vi "Impedance Excel Export.vi"(0 "template Path":path=path "C:/Users/L025200.LUXSHARE/Desktop/Released VNA Automatic 20150329/Templete/QSFP+_IBM.xls", 1 "Data Basic Path":path=path "S:/PNA_DATA/QSFP+  IBM 3m/Sample_#1_150331", 3 "Sheet Index List":i32[](array[numeric])=[1, 2, 3], 5 "Report  Path":path=path "S:/PNA_DATA/QSFP+  IBM 3m/Sample_#1_150331", 7 "error in (no error)":errorcluster caption="错误输入（无错误）") -> ()   [LabVIEW 2011]
uses:
  <vilib>/Utility/NIReport.llb/NI_report.lvclass
  <vilib>/Utility/file.llb/Read From Spreadsheet File (DBL).vi
  <vilib>/addons/_office/excel.llb/Excel Easy Table (num).vi
  <vilib>/Utility/NIReport.llb/Excel/NI_Excel.lvclass
  <vilib>/addons/_office/NI_ReportGenerationToolkit.lvlib
panel:
  in  "File Name":string=".txt"
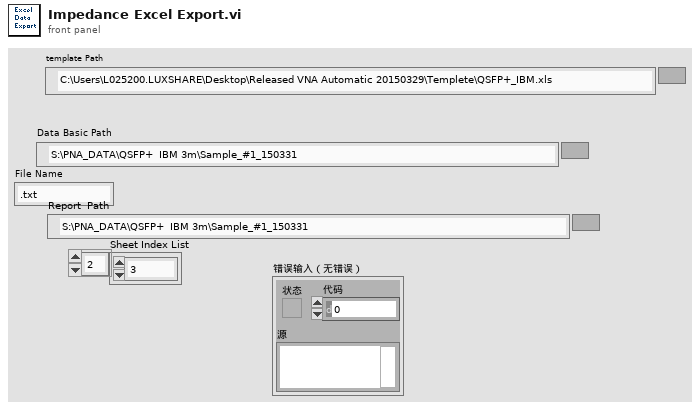
[diagram p1: front panel]
types:
  T1 = enum16{"Standard Report", "HTML", "Word", "Excel"}
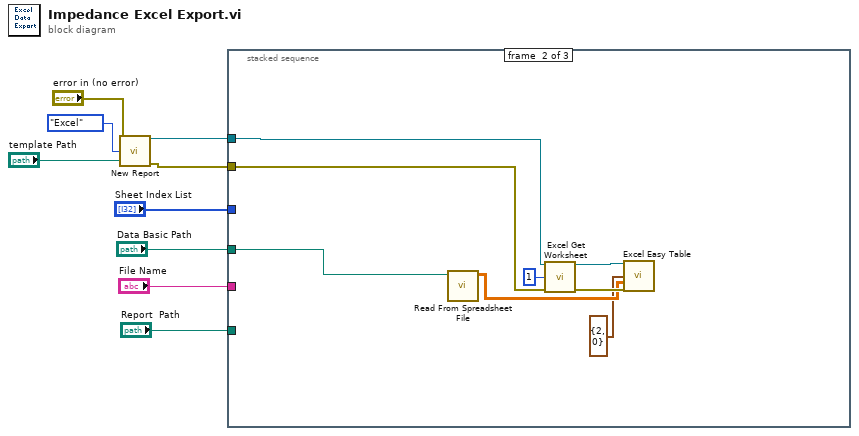
[diagram p0: block diagram]
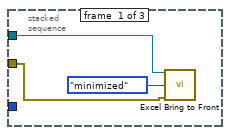
[diagram p2: hidden frame]
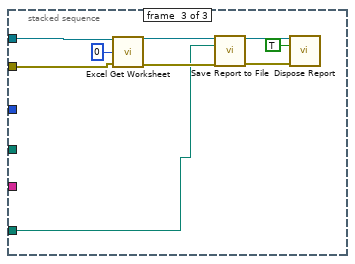
[diagram p3: hidden frame]
diagram:
  n1 = call <vilib>:"New Report.vi"("report type"=T1."Excel", "template (empty)"="template Path", "error in (no error)"="error in (no error)") -> ("report out"=w5:refnum<class "NI_report.lvclass">, "error out"=w3:errorcluster)  [unwired: 11 in]
  n2 = stacked-sequence {
    tunnel: "Data Basic Path" -> [_ w13 _]
    tunnel: "Sheet Index List" -> [_ _ _]
    tunnel: w5 -> [w11 w20 w29]
    tunnel: w3 -> [w10 w19 w22]
    tunnel: "File Name" -> [_ _ _]
    tunnel: "Report  Path" -> [_ _ w21]
    frame #0 {
      n3 = call <vilib>:"Excel Bring to Front.vi"("report in"=w11, "window state (maximized)"=enum16{"maximized", "minimized", "normal"}."minimized", "error in (no error)"=w10) -> ()  [unwired: 11 in, 2 out]
    }
    frame #1 {
      n4 = call-poly <vilib>:"Read From Spreadsheet File.vi"("file path (dialog if empty)"=w13) -> ("all rows"=w15:dbl[][])  [unwired: 6 in, 4 out]
      n5 = call <vilib>:"Excel Get Worksheet.vi"("report in"=w20, "worksheet index (0)"=1, "error in (no error)"=w19) -> ("report out"=w17:refnum<class "NI_report.lvclass">, "error out"=w18:errorcluster)  [unwired: 11 in]
      n6 = call-poly <vilib>:"Excel Easy Table.vi"("report in"=w17, "start (0, 0)"=cluster{"row":i32, "column":i32} {"row"=2, "column"=0}, "text data"=w15, "error in (no error)"=w18) -> ()  [unwired: 7 in, 5 out]
    }
    frame #2 {
      n7 = call <vilib>:"Excel Get Worksheet.vi"("report in"=w29, "worksheet index (0)"=0, "error in (no error)"=w22) -> ("report out"=w23:refnum<class "NI_report.lvclass">, "error out"=w24:errorcluster)  [unwired: 11 in]
      n8 = call-dynamic "Save Report to File.vi"("report in"=w23, "report file path"=w21, "error in (no error)"=w24) -> ("report out"=w26:refnum<class "NI_report.lvclass">, "error out"=w27:errorcluster)  [unwired: 11 in]
      n9 = call-dynamic "Dispose Report.vi"("report in"=w26, "wait until printing completed? (T)"=TRUE, "error in (no error)"=w27) -> ()  [unwired: 12 in, 1 out]
    }
  }
